vi "Refgroup.vi"(6 "Pane":refnum<vi>, 7 "Action":enum16{"GetRef", "ChkRef"}(ring)) -> (0 "AreaSize":T1, 1 "Ref_Gmsg":refnum<vi>, 2 "Ref_Ball":refnum<vi>, 3 "Ref_brick":refnum<vi>[](array[refnum]))   [LabVIEW 8.6]
uses:
  <vilib>/Utility/miscctls.llb/LVBoundsTypeDef.ctl
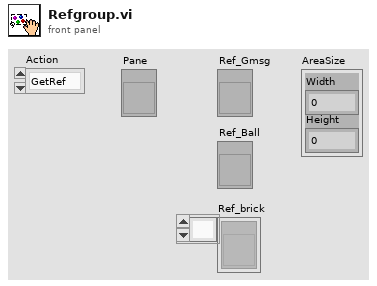
[diagram p1: front panel]
types:
  T1 = typedef "LVBoundsTypeDef.ctl" = cluster{"Width":u32, "Height":u32}
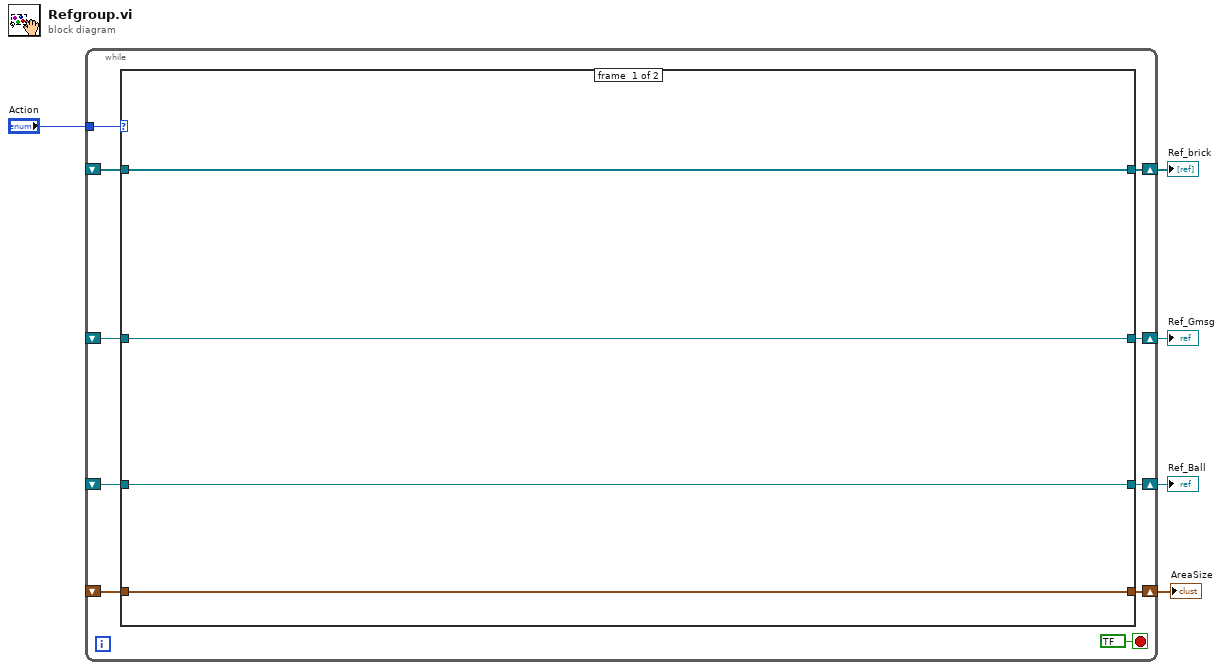
[diagram p0: block diagram]
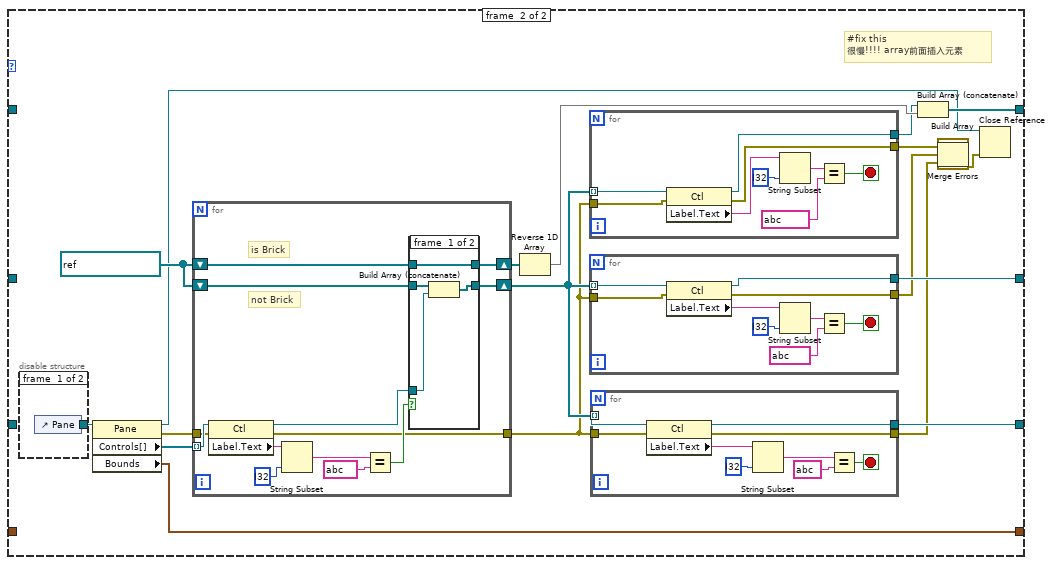
[diagram p2: hidden frame]
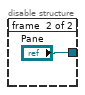
[diagram p3: hidden frame]
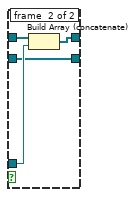
[diagram p4: hidden frame]
diagram:
  n1 = while {
    shift-right: [w12] -> w2
    shift-left: _ -> [w6]
    shift-right: [w15] -> w5
    shift-left: _ -> [w8]
    shift-right: [w14] -> w4
    shift-left: _ -> [w7]
    shift-right: [w13] -> w3
    shift-left: _ -> [w9]
    tunnel: "Action" -> [w10]
    stop <- bool ? stop-if-true
    n2 = case shown="\"ChkRef\"" w10 {
      tunnel: [w18 w36] -> w15
      tunnel: [w17 w35] -> w14
      tunnel: [w19 w34] -> w13
      tunnel: [w16 w33] -> w12
      tunnel: w9 -> [w19 _]
      tunnel: w8 -> [w18 _]
      tunnel: w7 -> [w17 _]
      tunnel: w6 -> [w16 _]
      frame #0 {
      }
      frame #1 {
        w32 = refnum<vi>[] ?
        # "#fix this\n很慢!!!! array前面插入元素"
        n3 = disable-structure shown="Enabled" {
          disable-tunnel: [w39 "Pane"] -> w38
          frame #0 {
            n4 = control-ref of="Pane"() -> (w39:refnum<vi>)
          }
          frame #1 {
          }
        }
        n5 = property class="Pane"(reference=w38) -> (reference out=w27:refnum<vi>, error out=w29:errorcluster, "Controls[]"=w31:refnum<vi>[], "Bounds"=w33:T1)  [unwired: 1 in]
        n6 = for {
          shift-right: [w75] -> w37
          shift-left: w32 -> [w76]
          tunnel: [w73] -> w28
          shift-right: [w71] -> w30
          shift-left: w32 -> [w70]
          tunnel: w31 -> [w69] mode=indexing
          tunnel: w29 -> [w68]
          # "not Brick"
          # "is Brick"
          n7 = property on="Property Node" class="Ctl"(reference=w69, error in=w68) -> (reference out=w72:refnum<vi>, error out=w73:errorcluster, "Label.Text"=w74:string)
          n8 = String Subset(string=w74, length (rest)=i32 ? ("length (rest)")) -> (substring=w78:string)  [unwired: 1 in]
          n9 = Equal?(x=w78, y=string ?) -> (x = y?=w77:bool)
          n10 = case shown="True" w77 {
            tunnel: w76 -> [w84 w87]
            tunnel: [w84 w88] -> w75
            tunnel: w72 -> [w83 w86]
            tunnel: [w82 w85] -> w71
            tunnel: w70 -> [w81 w85]
            frame #0 {
              n11 = Build Array (concatenate)(w81, w83) -> (w82:refnum<vi>[])
            }
            frame #1 {
              n12 = Build Array (concatenate)(w87, w86) -> (w88:refnum<vi>[])
            }
          }
        }
        n13 = Reverse 1D Array(array=w37) -> (reversed array=w22:refnum<vi>[])
        n14 = for {
          tunnel: [w45] -> w25
          tunnel: [w43] -> w21
          tunnel: w30 -> [w42] mode=indexing
          tunnel: w28 -> [w41]
          stop <- w44 stop-if-true
          n15 = property on="Property Node" class="Ctl"(reference=w42, error in=w41) -> (reference out=w43:refnum<vi>, error out=w45:errorcluster, "Label.Text"=w49:string)
          n16 = String Subset(string=w49, length (rest)=i32 ? ("length (rest)")) -> (substring=w48:string)  [unwired: 1 in]
          n17 = Equal?(x=w48, y=string ?) -> (x = y?=w44:bool)
        }
        n18 = for {
          tunnel: [w62] -> w36
          tunnel: [w61] -> w23
          tunnel: w30 -> [w60] mode=indexing
          tunnel: w28 -> [w59]
          stop <- w63 stop-if-true
          n19 = property on="Property Node" class="Ctl"(reference=w60, error in=w59) -> (reference out=w62:refnum<vi>, error out=w61:errorcluster, "Label.Text"=w67:string)
          n20 = String Subset(string=w67, length (rest)=i32 ? ("length (rest)")) -> (substring=w66:string)  [unwired: 1 in]
          n21 = Equal?(x=w66, y=string ?) -> (x = y?=w63:bool)
        }
        n22 = for {
          tunnel: [w54] -> w35
          tunnel: [w53] -> w24
          tunnel: w30 -> [w51] mode=indexing
          tunnel: w28 -> [w50]
          stop <- w52 stop-if-true
          n23 = property on="Property Node" class="Ctl"(reference=w51, error in=w50) -> (reference out=w54:refnum<vi>, error out=w53:errorcluster, "Label.Text"=w55:string)
          n24 = String Subset(string=w55, length (rest)=i32 ? ("length (rest)")) -> (substring=w56:string)  [unwired: 1 in]
          n25 = Equal?(x=w56, y=string ?) -> (x = y?=w52:bool)
        }
        n26 = Build Array (concatenate)(w21, w22) -> (w34:refnum<vi>[])
        n27 = Build Array(w25, w23, w24) -> (w20:errorcluster[])
        n28 = call <vilib>:"Merge Errors.vi"("error array in"=w20) -> ("error out"=w26:errorcluster)  [unwired: 6 in]
        n29 = Close Reference(reference=w27, error in (no error)=w26) -> ()  [unwired: 1 out]
      }
    }
  }
  "Ref_Gmsg" <- w5
  "Ref_Ball" <- w4
  "Ref_brick" <- w3
  "AreaSize" <- w2
